vi "总氮通讯.vi"() -> ()   [LabVIEW 2016, in "斯坦道总氮.lvlib"]
uses:
  <vilib>/Plasmionique/MB Master/MB_Master_TCP/MB_Master_TCP.lvclass
  C:/Program Files (x86)/National Instruments/LabVIEW 2016/vi.lib/Plasmionique/MB Master/MB_Master/MB_Master.lvclass
  <vilib>/NI/Modbus Library/API/Wrapper/Create TCP Slave.vi
  <vilib>/Utility/config.llb/Write Key (Boolean).vi
  <vilib>/Utility/config.llb/Write Key (String).vi
  <vilib>/Plasmionique/MB Master/MB_Master/MB_Master.lvclass
  <vilib>/NI/Modbus Library/API/slave/Modbus Slave.lvclass
  <vilib>/Utility/config.llb/NI_LVConfig.lvlib
  <vilib>/Plasmionique/MB Master/MB Master.lvlib
  <vilib>/NI/Modbus Library/API/Wrapper/API Main.lvlib
panel:
  out "总氮测量数据区":u16[](array[numeric])
  out "总氮状态告警区":u16[](array[numeric])
  out "总磷状态告警区":u16[](array[numeric])
  out "总磷测量数据区":u16[](array[numeric])
  out "序列号":string
  out "状态告警区":T1
  out "测量数据区":T2 {"单位" items=["ug/L", "mg/L", "ppm", "mg/m3", "cm", "ppb", "ug/m3", "%", "nmol/mol", "umol/mol", "MPN/L", "MPN/100ml", "ng/m3", "NTU", "无量纲", "ms/cm", "us/cm", "℃", "mV", "万个/L"]}
  out "status":bool
  out "关键参数区":T3
  in  "读关键参数区":bool
  in  "读状态告警区":bool
  in  "读测量数据区":bool
  in  "站号":u16(ring) items=["总磷"=1, "氨氮"=3]
  in  "停止":bool
  in  "启动":bool
  in  "控制命令":u16(ring) items=["启动测量"=1, "标样核查"=2, "零点核查"=3, "跨度核查"=4, "空白测试"=5, "平行样测试"=6, "加标回收"=7, "空白校准"=8, "标样校准"=9, "初始化（清洗）"=10, "停止测试"=11, "仪器重启"=12, "校时"=13, "模式设置"=14, "测量间隔设置"=15]
  in  "控制命令参数":u16[](array[numeric]) format="%04xH"
  in  "VISA Resource":refnum<visa-resource-name>
  in  "启用模块":bool
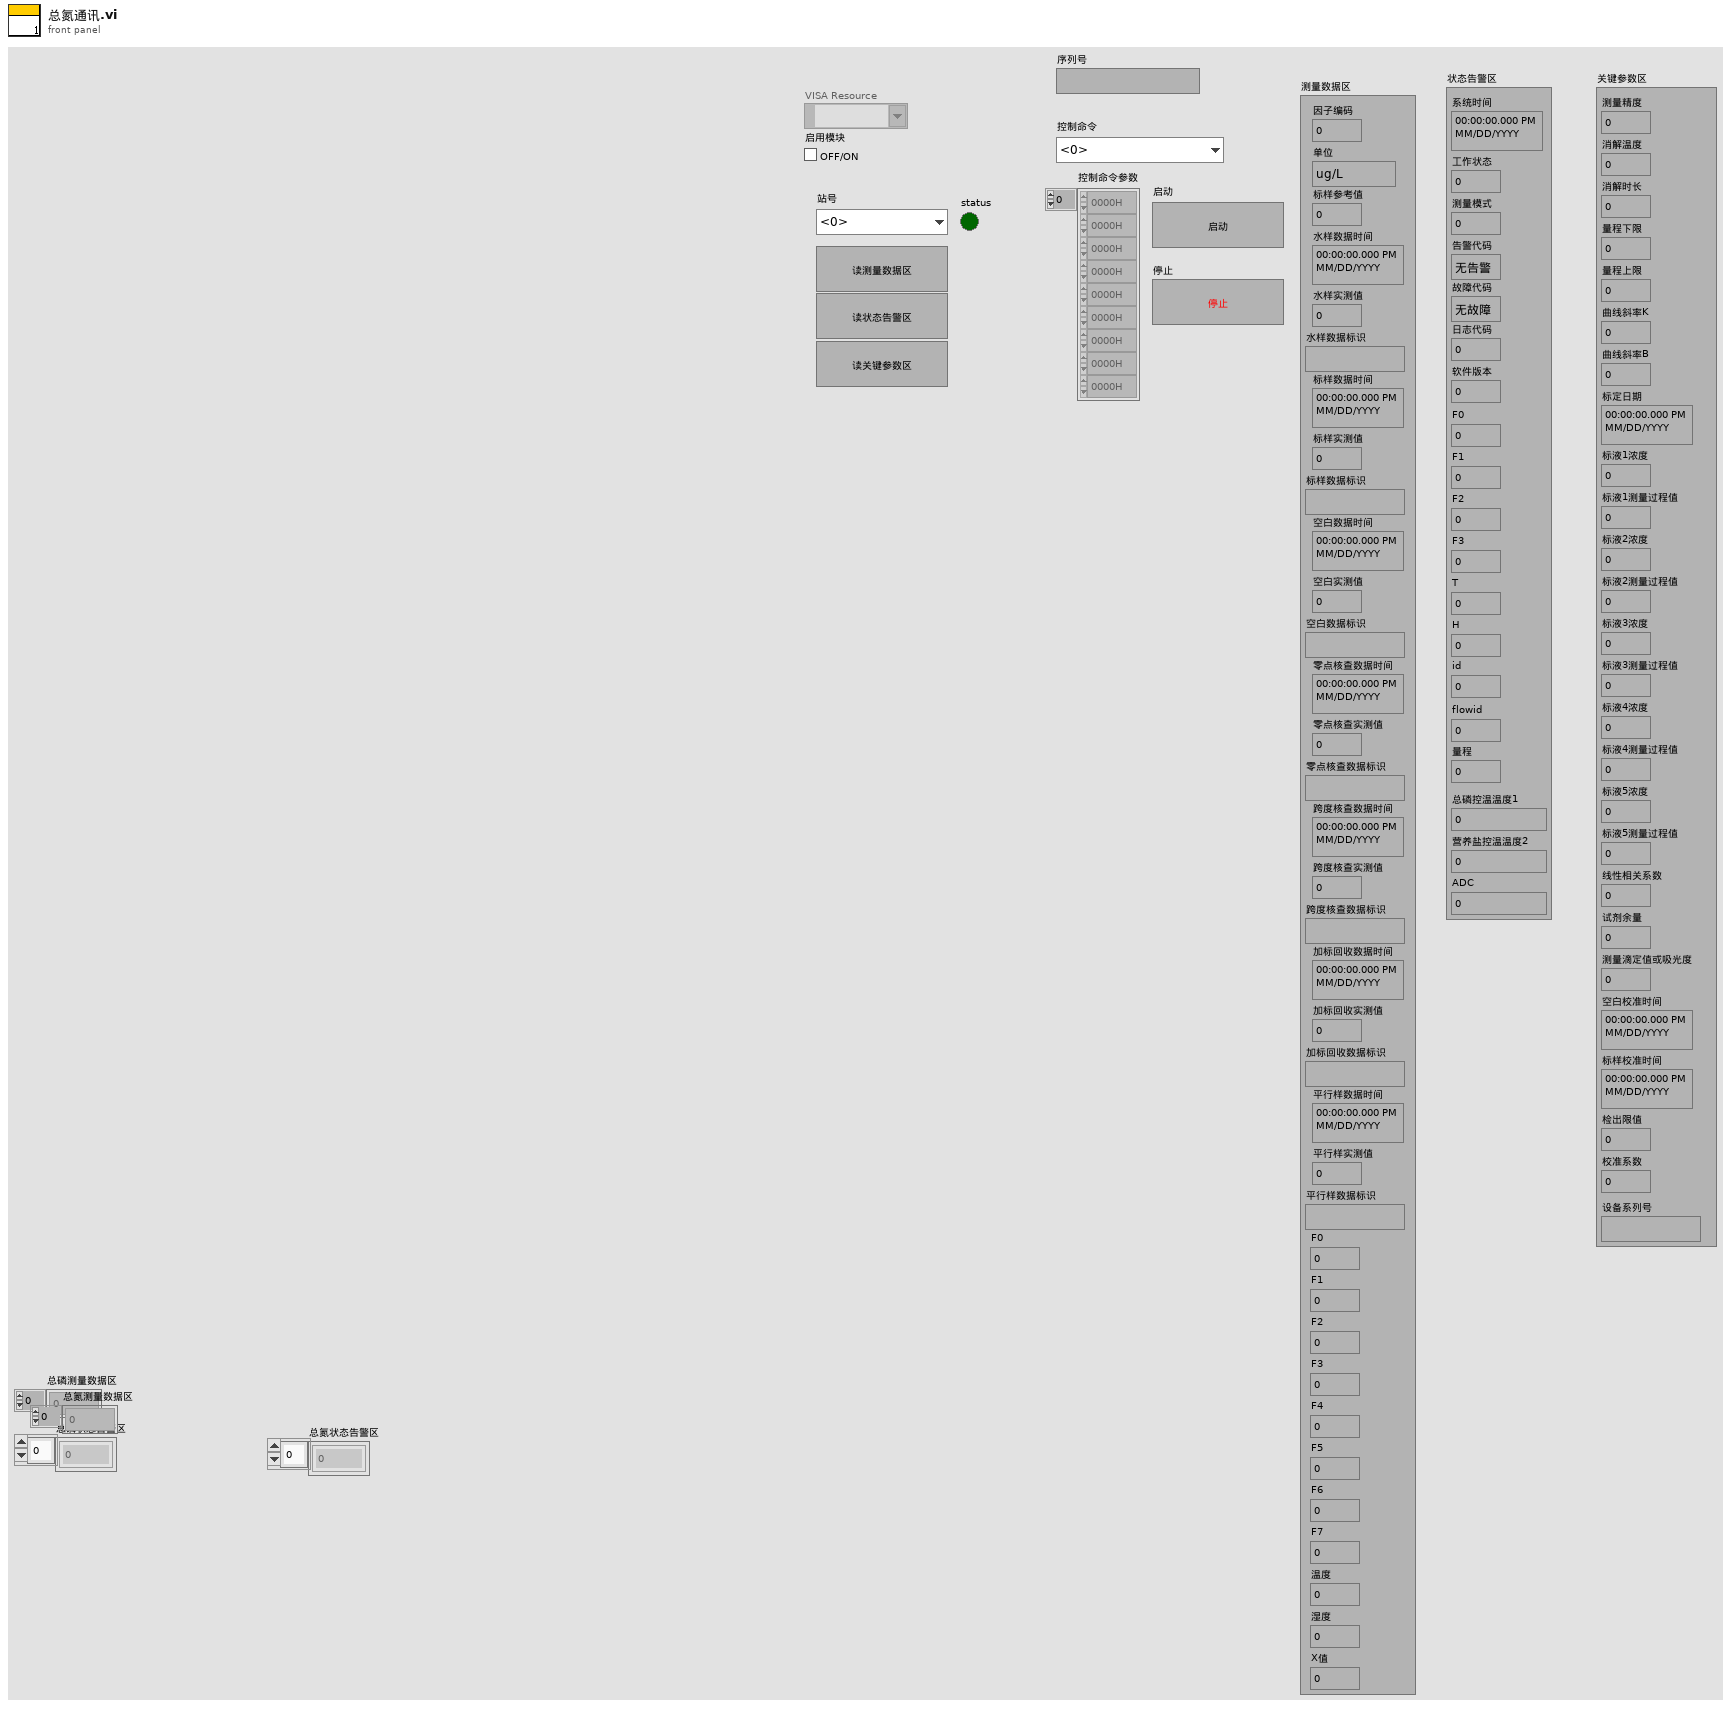
[diagram p1: front panel]
types:
  T1 = cluster{"系统时间":timestamp, "工作状态":u16, "测量模式":u16, "告警代码":enum16{"无告警", "缺试剂告警", "缺水样告警", "缺蒸馏水告警", "缺标液告警", "仪表漏液告警", "标定异常告警", "超量程告警", "加热异常", "低试剂预警", "超上限告警", "超下限告警", "仪表内部其他异常", "滴定异常告警", "电极异常告警", "量程切换告警", "参数设置告警", "PH电极电位异常", "电导率电极异常", "浊度光度异常", "溶解氧电极异常", "溶解氧光强异常", "温度异常告警", "PH异常告警", "溶解氧异常告警", "电导率异常告警", "浊度异常告警", "叶绿素异常告警", "藻密度异常告警", "蓝绿藻异常告警", "ORP异常告警", "氨氮异常告警", "清洁刷异常告警", "SD卡异常告警", "蓝牙异常告警", "Wifi异常告警", "流程异常告警"}, "故障代码":enum16{"无故障", "电机故障", "温度故障", "通讯故障", "滴定故障"}, "日志代码":u16, "软件版本":u16, "F0":sgl, "F1":sgl, "F2":sgl, "F3":sgl, "T":sgl, "H":sgl, "id":u16, "flowid":u16, "量程":u16, "总磷控温温度1":sgl, "营养盐控温温度2":sgl, "ADC":sgl}
  T2 = cluster{"因子编码":u32, "单位":u16, "标样参考值":sgl, "水样数据时间":timestamp, "水样实测值":sgl, "水样数据标识":string, "标样数据时间":timestamp, "标样实测值":sgl, "标样数据标识":string, "空白数据时间":timestamp, "空白实测值":sgl, "空白数据标识":string, "零点核查数据时间":timestamp, "零点核查实测值":sgl, "零点核查数据标识":string, "跨度核查数据时间":timestamp, "跨度核查实测值":sgl, "跨度核查数据标识":string, "加标回收数据时间":timestamp, "加标回收实测值":sgl, "加标回收数据标识":string, "平行样数据时间":timestamp, "平行样实测值":sgl, "平行样数据标识":string, "F0":sgl, "F1":sgl, "F2":sgl, "F3":sgl, "F4":sgl, "F5":sgl, "F6":sgl, "F7":sgl, "温度":sgl, "湿度":sgl, "X值":sgl}
  T3 = cluster{"测量精度":u16, "消解温度":u16, "消解时长":u16, "量程下限":sgl, "量程上限":sgl, "曲线斜率K":sgl, "曲线斜率B":sgl, "标定日期":timestamp, "标液1浓度":sgl, "标液1测量过程值":sgl, "标液2浓度":sgl, "标液2测量过程值":sgl, "标液3浓度":sgl, "标液3测量过程值":sgl, "标液4浓度":sgl, "标液4测量过程值":sgl, "标液5浓度":sgl, "标液5测量过程值":sgl, "线性相关系数":sgl, "试剂余量":u32, "测量滴定值或吸光度":sgl, "空白校准时间":timestamp, "标样校准时间":timestamp, "检出限值":sgl, "校准系数":sgl, "设备系列号":string}
  T4 = typedef "NI_LVConfig.lvlib/Config Data RefNum.ctl" = refnum<k1>
  T5 = enum8{"Enabled", "Disabled", "Disabled and Grayed Out"}
  T6 = cluster{"系统时间":timestamp, "工作状态":enum16{"空闲", "水样测试", "标样核查", "零点核查", "跨度核查", "空白测试", "平行样测试", "加标回收", "空白校准", "标样校准", "初始化（清洗）"}, "测量模式":enum16{"待机", "连续模式", "周期模式", "定点模式", "受控模式", "手动模式"}, "告警代码":enum16{"无告警", "缺试剂告警", "缺水样告警", "缺蒸馏水告警", "缺标液告警", "仪表漏液告警", "标定异常告警", "超量程告警", "加热异常", "低试剂预警", "超上限告警", "超下限告警", "仪表内部其他异常", "滴定异常告警", "电极异常告警", "量程切换告警", "参数设置告警", "PH电极电位异常", "电导率电极异常", "浊度光度异常", "溶解氧电极异常", "溶解氧光强异常", "温度异常告警", "PH异常告警", "溶解氧异常告警", "电导率异常告警", "浊度异常告警", "叶绿素异常告警", "藻密度异常告警", "蓝绿藻异常告警", "ORP异常告警", "氨氮异常告警", "清洁刷异常告警", "SD卡异常告警", "蓝牙异常告警", "Wifi异常告警", "流程异常告警"}, "故障代码":enum16{"无故障", "电机故障", "温度故障", "通讯故障", "滴定故障"}, "日志代码":u16, "软件版本":u16, "F0":sgl, "F1":sgl, "F2":sgl, "F3":sgl, "T":sgl, "H":sgl, "id":u16, "flowid":u16, "量程":u16, "总磷控温温度1":sgl, "营养盐控温温度2":sgl, "ADC":sgl}
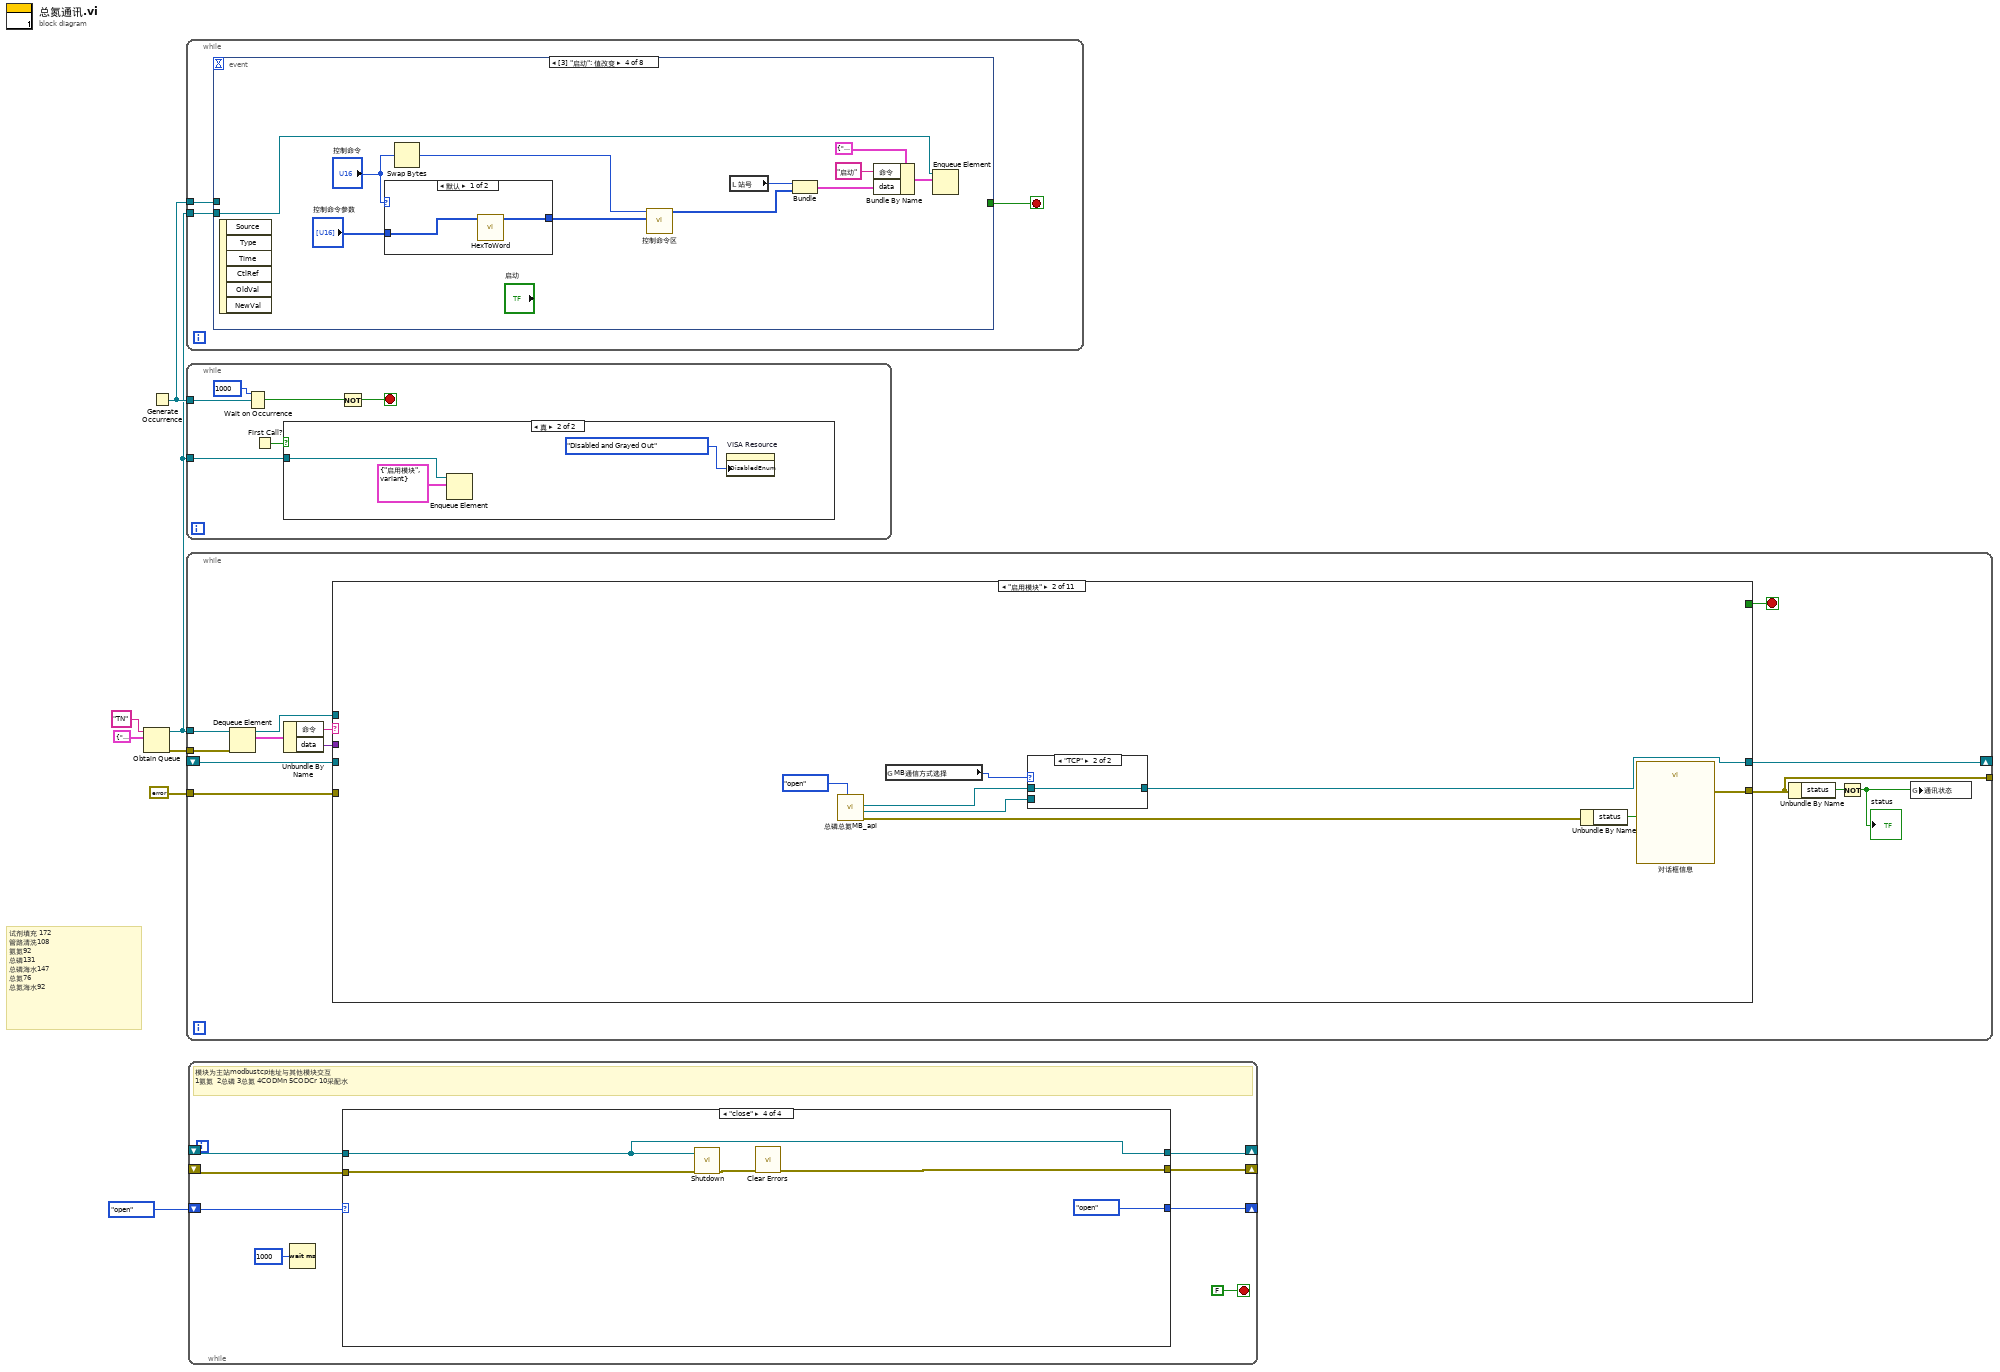
[diagram p0: block diagram]
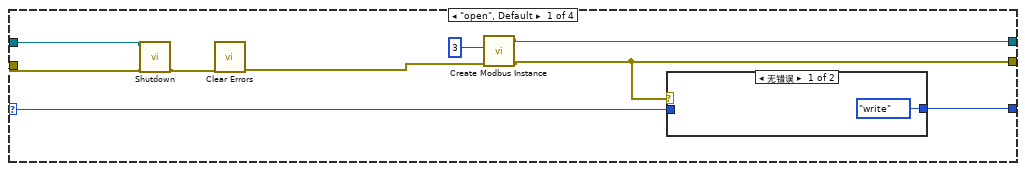
[diagram p2: hidden frame]
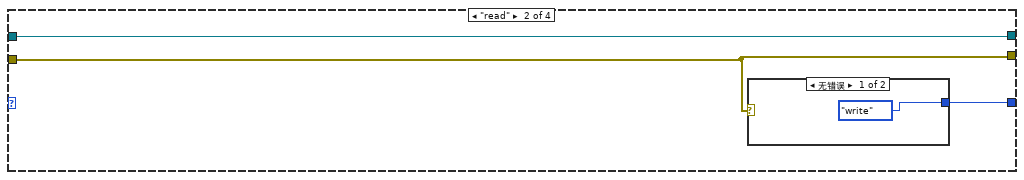
[diagram p4: hidden frame]
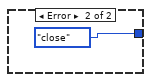
[diagram p5: hidden frame]
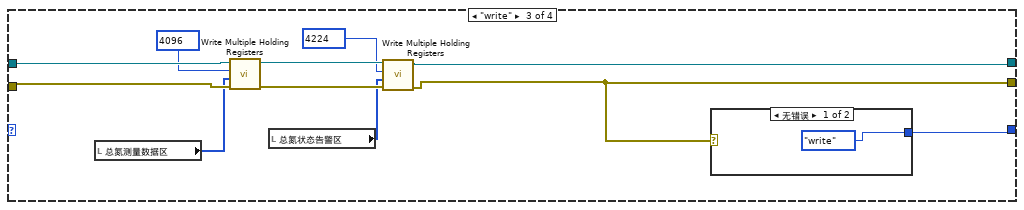
[diagram p6: hidden frame]
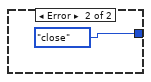
[diagram p7: hidden frame]
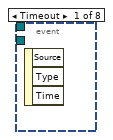
[diagram p9: hidden frame]
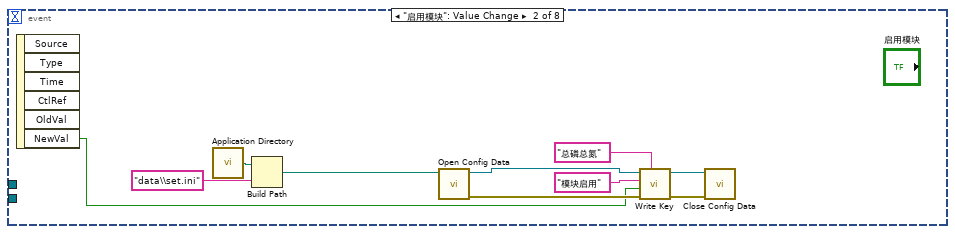
[diagram p10: hidden frame]
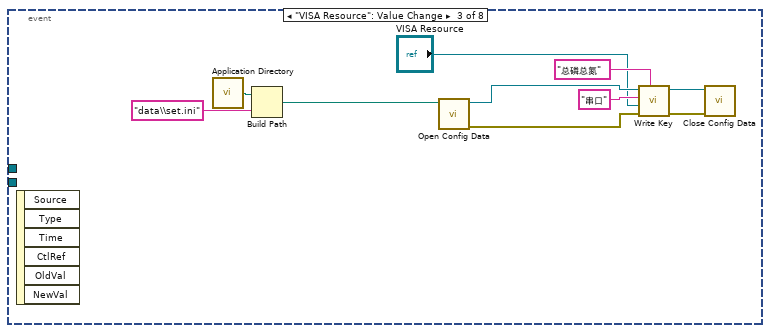
[diagram p11: hidden frame]
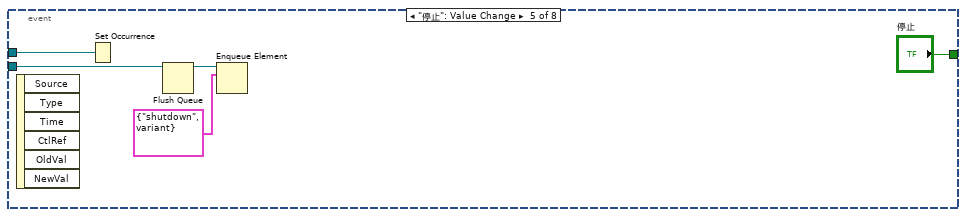
[diagram p13: hidden frame]
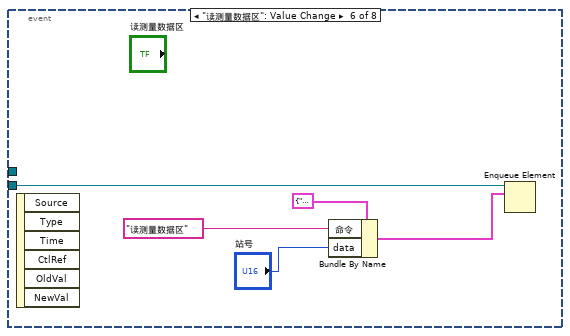
[diagram p14: hidden frame]
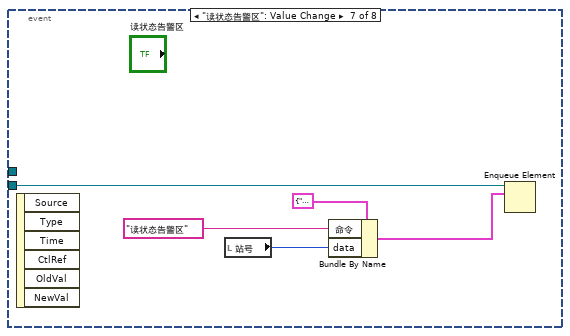
[diagram p15: hidden frame]
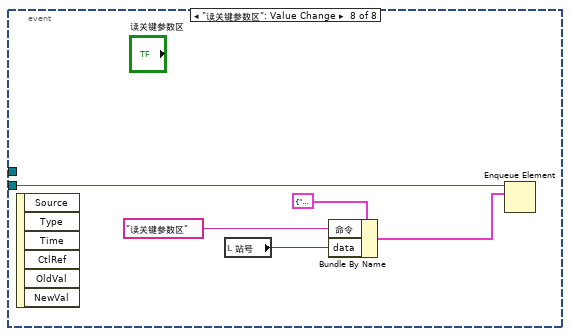
[diagram p16: hidden frame]
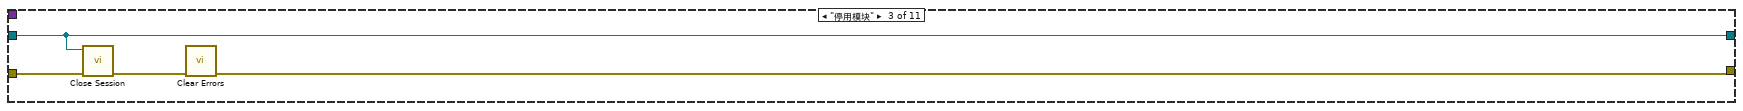
[diagram p19: hidden frame]
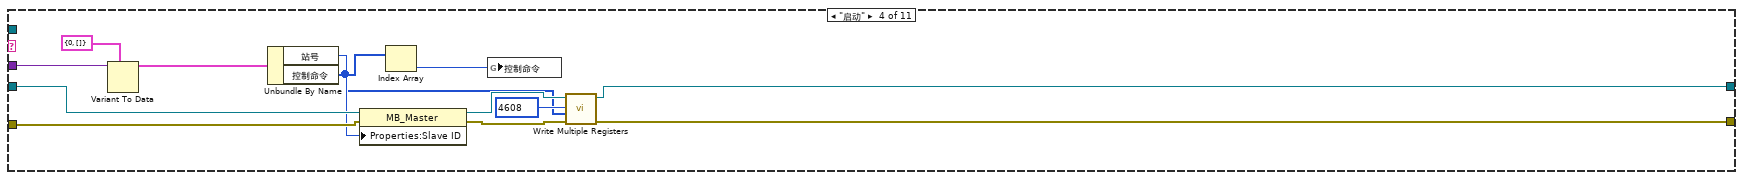
[diagram p20: hidden frame]
diagram:
  # "试剂填充 172 \n管路清洗108\n氨氮92\n总磷131\n总磷海水147\n总氮76\n总氮海水92"
  n1 = Obtain Queue(name (unnamed)="TN" ("名称（未命名）"), element data type=cluster{"命令":string, "data":variant} {"命令"="", "data"=variant}) -> (queue out=w2:refnum<queue>, error out=w5:errorcluster)  [unwired: 3 in, 1 out]
  n2 = Generate Occurrence() -> (w3:refnum<k4>)
  n3 = while {
    tunnel: w2 -> [w10]
    tunnel: w3 -> [w8]
    stop <- w9 stop-if-true
    n4 = event shown="[3] \"启动\": 值改变" {
      selector: _ -> [_ _ _ _ _ _ _ _]
      dyn-events: _ -> [_ _ _ _ _ _ _ _]
      timeout: _ -> [_ _ _ _ _ _ _ _]
      tunnel: w10 -> [_ _ _ w41 w48 w54 w59 w64]
      tunnel: [_ _ _ _ "停止" _ _ _] -> w9
      tunnel: w8 -> [_ _ _ _ w45 _ _ _]
      event Timeout {
        n5 = event-data() -> ()  [unwired: 1 in, 3 out]
      }
      event "启用模块": Value Change {
        n6 = event-data() -> ("NewVal"=w11:bool)  [unwired: 1 in, 5 out]
        n7 = call <vilib>:"Application Directory.vi"() -> ("Application Directory"=w13:path)
        n8 = Build Path(base path=w13, name or relative path="data\\set.ini" ("名称或相对路径")) -> (appended path=w14:path)
        n9 = call <vilib>:"Open Config Data.vi"("configuration file path"=w14) -> ("error out"=w20:errorcluster, "refnum"=w19:T4)  [unwired: 8 in, 1 out]
        n10 = call-poly <vilib>:"Write Key.vi"("section"="总磷总氮", "error in (no error)"=w20, "value"=w11, "key"="模块启用", "refnum"=w19) -> ("error out"=w16:errorcluster, "refnum out"=w12:T4)  [unwired: 4 in, 1 out]
        n11 = call <vilib>:"Close Config Data.vi"("error in (no error)"=w16, "refnum"=w12) -> ()  [unwired: 8 in, 2 out]
      }
      event "VISA Resource": Value Change {
        n12 = event-data() -> ()  [unwired: 1 in, 6 out]
        n13 = call <vilib>:"Application Directory.vi"() -> ("Application Directory"=w23:path)
        n14 = Build Path(base path=w23, name or relative path="data\\set.ini" ("名称或相对路径")) -> (appended path=w24:path)
        n15 = call <vilib>:"Open Config Data.vi"("configuration file path"=w24) -> ("error out"=w30:errorcluster, "refnum"=w29:T4)  [unwired: 8 in, 1 out]
        n16 = call-poly <vilib>:"Write Key.vi"("section"="总磷总氮", "error in (no error)"=w30, "value"="VISA Resource", "key"="串口", "refnum"=w29) -> ("error out"=w26:errorcluster, "refnum out"=w22:T4)  [unwired: 4 in, 1 out]
        n17 = call <vilib>:"Close Config Data.vi"("error in (no error)"=w26, "refnum"=w22) -> ()  [unwired: 8 in, 2 out]
      }
      event "启动": Value Change {
        n18 = event-data() -> ()  [unwired: 1 in, 6 out]
        n19 = case shown="默认" "控制命令" {
          tunnel: "控制命令参数" -> [w43 w44]
          tunnel: [w42 w44] -> w31
          frame Default {
            n20 = call "HexToWord.vi"("数组"=w43) -> ("WORD"=w42:u16[])  [unwired: 10 in]
          }
          frame 13 {
          }
        }
        n21 = Swap Bytes(anything="控制命令") -> (byte swapped=w34:u16)
        n22 = call "控制命令区.vi"("控制命令参数"=w31, "控制命令"=w34) -> ("控制命令"=w37:u16[])  [unwired: 9 in]
        n23 = local read "站号"() -> (w36:u16)
        n24 = Bundle("站号"=w36, "控制命令"=w37) -> (w35:cluster{"站号":u16, "控制命令":u16[]})  [unwired: 1 in]
        n25 = Bundle By Name(cluster=cluster{"命令":string, "data":variant} {"命令"="", "data"=variant} ("元素"), "命令"="启动", "data"=w35) -> (w39:cluster{"命令":string, "data":variant})
        n26 = Enqueue Element(queue=w41, element=w39) -> ()  [unwired: 2 in, 3 out]
      }
      event "停止": Value Change {
        n27 = event-data() -> ()  [unwired: 1 in, 6 out]
        n28 = Set Occurrence(w45) -> ()
        n29 = Flush Queue(queue=w48) -> (queue out=w47:refnum<queue>)  [unwired: 1 in, 2 out]
        n30 = Enqueue Element(queue=w47, element=cluster{"命令":string, "data":variant} {"命令"="shutdown", "data"=variant} ("元素")) -> ()  [unwired: 2 in, 3 out]
      }
      event "读测量数据区": Value Change {
        n31 = event-data() -> ()  [unwired: 1 in, 6 out]
        n32 = Bundle By Name(cluster=cluster{"命令":string, "data":variant} {"命令"="", "data"=variant} ("元素"), "命令"="读测量数据区", "data"="站号") -> (w52:cluster{"命令":string, "data":variant})
        n33 = Enqueue Element(queue=w54, element=w52) -> ()  [unwired: 2 in, 3 out]
      }
      event "读状态告警区": Value Change {
        n34 = event-data() -> ()  [unwired: 1 in, 6 out]
        n35 = local read "站号"() -> (w55:u16)
        n36 = Bundle By Name(cluster=cluster{"命令":string, "data":variant} {"命令"="", "data"=variant} ("元素"), "命令"="读状态告警区", "data"=w55) -> (w57:cluster{"命令":string, "data":variant})
        n37 = Enqueue Element(queue=w59, element=w57) -> ()  [unwired: 2 in, 3 out]
      }
      event "读关键参数区": Value Change {
        n38 = event-data() -> ()  [unwired: 1 in, 6 out]
        n39 = local read "站号"() -> (w60:u16)
        n40 = Bundle By Name(cluster=cluster{"命令":string, "data":variant} {"命令"="", "data"=variant} ("元素"), "命令"="读关键参数区", "data"=w60) -> (w62:cluster{"命令":string, "data":variant})
        n41 = Enqueue Element(queue=w64, element=w62) -> ()  [unwired: 2 in, 3 out]
      }
    }
  }
  n42 = while {
    tunnel: w3 -> [w70]
    tunnel: w2 -> [w66]
    stop <- w67 stop-if-true
    n43 = Wait on Occurrence(2:w70, 3:1000 ("毫秒超时(-1)")) -> (0:w68:bool)  [unwired: 1 in]
    n44 = First Call?() -> (First Call?: T/F=w65:bool)
    n45 = case shown="真" w65 {
      tunnel: w66 -> [_ w72]
      frame False {
      }
      frame True {
        n46 = Enqueue Element(queue=w72, element=cluster{"命令":string, "data":variant} {"命令"="启用模块", "data"=variant} ("元素")) -> ()  [unwired: 2 in, 3 out]
        n47 = property on="VISA Resource" class="VISAName"("DisabledEnum"=T5."Disabled and Grayed Out" ("禁用")) -> ()  [unwired: 2 in, 2 out]
      }
    }
    n48 = Not(x=w68) -> (.not. x?=w67:bool)
  }
  n49 = while {
    tunnel: w2 -> [w86]
    tunnel: w5 -> [w85]
    shift-right: [w83] -> _
    shift-left: _ -> [w82]
    tunnel: errorcluster {"status"=FALSE, "code"=0, "source"=""} ("error out") -> [w81]
    tunnel: [w76] -> _
    stop <- w84 stop-if-true
    n50 = Dequeue Element(queue=w86, error in (no error)=w85) -> (queue out=w77:refnum<queue>, element=w79:cluster{"命令":string, "data":variant})  [unwired: 1 in, 2 out]
    n51 = Unbundle By Name(w79) -> ("命令"=w80:string, "data"=w78:variant)
    n52 = case shown="\"启用模块\"" w80 {
      tunnel: w78 -> [_ _ _ w112 w123 w140 w150 w164 w182 w196 _]
      tunnel: w77 -> [_ _ _ _ _ _ _ _ _ _ w209]
      tunnel: [_ _ _ _ _ _ _ _ _ _ TRUE] -> w84
      tunnel: [w87 w89 w99 w115 w126 w142 w154 w173 w189 w203 w205] -> w83
      tunnel: [w88 w95 w100 w114 w125 w141 w155 w163 w190 w204 w206] -> w76
      tunnel: w82 -> [w87 _ w99 w111 w122 w139 w149 w167 w185 w199 w205]
      tunnel: w81 -> [w88 _ w102 w108 w119 w136 w147 w168 w186 w200 w207]
      frame Default {
      }
      frame "启用模块" {
        n53 = call "总磷总氮MB_api.vi"("STEP"=enum16{"open", "read", "write", "close"}."open") -> ("error out"=w93:errorcluster, "MB session out"=w90:refnum<class "MB_Master.lvclass">, "MB_TCP session"=w91:refnum<class "MB_Master_TCP.lvclass">)  [unwired: 7 in, 1 out]
        n54 = global read "总氮断电保存全局变量.vi" "MB通信方式选择"() -> (w92:enum16{"串口", "TCP"})
        n55 = case shown="\"TCP\"" w92 {
          tunnel: w91 -> [_ w98]
          tunnel: w90 -> [w97 _]
          tunnel: [w97 w98] -> w89
          frame "串口", Default {
          }
          frame "TCP" {
          }
        }
        n56 = Unbundle By Name(w93) -> ("status"=w96:bool)
        n57 = call "对话框信息"("Enable"=w96) -> ("error out"=w95:errorcluster)  [unwired: 9 in, 1 out]
      }
      frame "停用模块" {
        n58 = call-dynamic "Close Session.vi"("error in (no error)"=w102, "MB session in"=w99) -> ("error out"=w101:errorcluster)  [unwired: 9 in]
        n59 = call <vilib>:"Clear Errors.vi"("error in (no error)"=w101) -> ("error out"=w100:errorcluster)  [unwired: 5 in, 1 out]
      }
      frame "启动" {
        n60 = Variant To Data(type=cluster{"站号":u16, "控制命令":u16[]} {"站号"=0, "控制命令"=[]} ("输出簇"), Variant=w112) -> (data=w106:cluster{"站号":u16, "控制命令":u16[]})  [unwired: 1 in, 1 out]
        n61 = Unbundle By Name(w106) -> ("站号"=w105:u16, "控制命令"=w103:u16[])
        n62 = property class="MB_Master"(reference=w111, error in=w108, "Properties:Slave ID"=w105) -> (reference out=w110:refnum<class "MB_Master.lvclass">, error out=w109:errorcluster)
        n63 = Index Array(array=w103) -> (element=w104:u16)  [unwired: 1 in]
        n64 = global write "VAR总氮全局变量.vi" "控制命令"(w104) -> ()
        n65 = call <vilib>:"Write Multiple Registers.vi"("error in (no error)"=w109, "values"=w103, "starting address"=u16 4608, "MB session in"=w110) -> ("error out"=w114:errorcluster, "MB session out"=w115:refnum<class "MB_Master.lvclass">)  [unwired: 6 in]
      }
      frame "盲样测试" {
        n66 = Variant To Data(type=0, Variant=w123) -> (data=w116:i32)  [unwired: 1 in, 1 out]
        n67 = case shown="默认" w116 {
          tunnel: [u16[] [] ("values") u16[] [33539, 0] ("values") u16[] [23555, 0] ("values")] -> w118
          frame Default {
          }
          frame 1 {
            # "总磷盲样测试命令"
          }
          frame 3 {
            # "氨氮盲样测试"
          }
        }
        n68 = property class="MB_Master"(reference=w122, error in=w119, "Properties:Slave ID"=w116) -> (reference out=w121:refnum<class "MB_Master.lvclass">, error out=w120:errorcluster)
        n69 = call <vilib>:"Write Multiple Registers.vi"("error in (no error)"=w120, "values"=w118, "starting address"=u16 24592, "MB session in"=w121) -> ("error out"=w125:errorcluster, "MB session out"=w126:refnum<class "MB_Master.lvclass">)  [unwired: 6 in]
      }
      frame "debug" {
        n70 = Variant To Data(type=cluster{"站号":u16, "控制命令":u16[]} {"站号"=0, "控制命令"=[]} ("输出簇"), Variant=w140) -> (data=w134:cluster{"站号":u16, "控制命令":u16[]})  [unwired: 1 in, 1 out]
        n71 = Unbundle By Name(w134) -> ("站号"=w133:u16, "控制命令"=w131:u16[])
        n72 = property class="MB_Master"(reference=w139, error in=w136, "Properties:Slave ID"=w133) -> (reference out=w138:refnum<class "MB_Master.lvclass">, error out=w137:errorcluster)
        n73 = Index Array(array=w131) -> (element=w132:u16)  [unwired: 1 in]
        n74 = global write "VAR总氮全局变量.vi" "控制命令"(w132) -> ()
        n75 = call <vilib>:"Write Multiple Registers.vi"("error in (no error)"=w137, "values"=w131, "starting address"=u16 24594, "MB session in"=w138) -> ("error out"=w141:errorcluster, "MB session out"=w142:refnum<class "MB_Master.lvclass">)  [unwired: 6 in]
      }
      frame "读测量数据区" {
        n76 = Variant To Data(type=u8 1 ("Slave ID"), Variant=w150) -> (data=w145:u8)  [unwired: 1 in, 1 out]
        n77 = property class="MB_Master"(reference=w149, error in=w147, "Properties:Slave ID"=w145) -> (reference out=w148:refnum<class "MB_Master.lvclass">, error out=w146:errorcluster)
        n78 = call <vilib>:"Read Holding Registers.vi"("error in (no error)"=w146, "quantity"=u16 104, "starting address"=u16 4096, "MB session in"=w148) -> ("error out"=w155:errorcluster, "Registers"=w144:u16[], "MB session out"=w154:refnum<class "MB_Master.lvclass">)  [unwired: 5 in]
        n79 = call "测量数据区.vi"("数组"=w144) -> ("测量数据区"=w143:T2)  [unwired: 10 in]
        "测量数据区" <- w143
        n80 = case shown="2" w145 {
          tunnel: w143 -> [_ w156 w158]
          tunnel: w144 -> [_ w157 w159]
          frame 0, Default {
          }
          frame 1 {
            n81 = global write "VAR总氮全局变量.vi" "总磷测量数据区"(w156) -> ()
            "总磷测量数据区" <- w157
          }
          frame 2 {
            n82 = global write "VAR总氮全局变量.vi" "总氮测量数据区"(w158) -> ()
            "总氮测量数据区" <- w159
          }
        }
        n83 = global write "VAR总氮全局变量.vi" "测量数据区"(w143) -> ()
      }
      frame "读状态告警区" {
        n84 = Variant To Data(type=u8 1 ("Slave ID"), Variant=w164) -> (data=w169:u8)  [unwired: 1 in, 1 out]
        n85 = property class="MB_Master"(reference=w167, error in=w168, "Properties:Slave ID"=w169) -> (reference out=w166:refnum<class "MB_Master.lvclass">, error out=w165:errorcluster)
        n86 = call <vilib>:"Read Holding Registers.vi"("error in (no error)"=w165, "quantity"=u16 29, "starting address"=u16 4224, "MB session in"=w166) -> ("error out"=w163:errorcluster, "Registers"=w160:u16[], "MB session out"=w173:refnum<class "MB_Master.lvclass">)  [unwired: 5 in]
        n87 = call "状态告警区.vi"("数组"=w160) -> ("状态告警区"=w161:T6)  [unwired: 10 in]
        "状态告警区" <- w161
        n88 = global write "VAR总氮全局变量.vi" "状态告警区"(w161) -> ()
        n89 = Unbundle By Name(w161) -> ("id"=w162:u16)
        n90 = case shown="2, 76" w162 {
          tunnel: w161 -> [_ w174 w176]
          tunnel: w160 -> [_ w175 w177]
          frame 0, Default {
          }
          frame 1, 131 {
            n91 = global write "VAR总氮全局变量.vi" "总磷状态告警区"(w174) -> ()
            "总磷状态告警区" <- w175
          }
          frame 2, 76 {
            n92 = global write "VAR总氮全局变量.vi" "总氮状态告警区"(w176) -> ()
            "总氮状态告警区" <- w177
          }
        }
      }
      frame "读关键参数区" {
        n93 = Variant To Data(type=u8 1 ("Slave ID"), Variant=w182) -> (data=w180:u8)  [unwired: 1 in, 1 out]
        n94 = property class="MB_Master"(reference=w185, error in=w186, "Properties:Slave ID"=w180) -> (reference out=w184:refnum<class "MB_Master.lvclass">, error out=w183:errorcluster)
        n95 = call <vilib>:"Read Holding Registers.vi"("error in (no error)"=w183, "quantity"=u16 19, "starting address"=u16 4256, "MB session in"=w184) -> ("error out"=w190:errorcluster, "Registers"=w179:u16[], "MB session out"=w189:refnum<class "MB_Master.lvclass">)  [unwired: 5 in]
        n96 = call "关键参数区.vi"("数组"=w179) -> ("关键参数区"=w178:T3)  [unwired: 10 in]
        "关键参数区" <- w178
        n97 = global write "VAR总氮全局变量.vi" "关键参数区"(w178) -> ()
      }
      frame "读序列号" {
        n98 = Variant To Data(type=u8 1 ("Slave ID"), Variant=w196) -> (data=w194:u8)  [unwired: 1 in, 1 out]
        n99 = property class="MB_Master"(reference=w199, error in=w200, "Properties:Slave ID"=w194) -> (reference out=w198:refnum<class "MB_Master.lvclass">, error out=w197:errorcluster)
        n100 = call <vilib>:"Read Holding Registers.vi"("error in (no error)"=w197, "quantity"=u16 6, "starting address"=u16 3, "MB session in"=w198) -> ("error out"=w204:errorcluster, "Registers"=w193:u16[], "MB session out"=w203:refnum<class "MB_Master.lvclass">)  [unwired: 5 in]
        n101 = call "HexToString.vi"("数组"=w193) -> ("STRING"=w192:string[])  [unwired: 10 in]
        n102 = Index Array(array=w192) -> (element=w191:string)  [unwired: 1 in]
        "序列号" <- w191
        n103 = global write "VAR总氮全局变量.vi" "序列号"(w191) -> ()
      }
      frame "shutdown" {
        n104 = call-dynamic "Close Session.vi"("error in (no error)"=w207, "MB session in"=w205) -> ("error out"=w206:errorcluster)  [unwired: 9 in]
        n105 = Flush Queue(queue=w209) -> (queue out=w208:refnum<queue>)  [unwired: 1 in, 2 out]
        n106 = Release Queue(queue=w208) -> ()  [unwired: 2 in, 3 out]
      }
    }
    n107 = Unbundle By Name(w76) -> ("status"=w75:bool)
    n108 = Not(x=w75) -> (.not. x?=w74:bool)
    "status" <- w74
    n109 = global write "VAR总氮全局变量.vi" "通讯状态"(w74) -> ()
  }
  n110 = while {
    shift-right: [w216] -> _
    shift-left: _ -> [w218]
    shift-right: [w215] -> _
    shift-left: _ -> [w217]
    shift-right: [w212] -> _
    shift-left: enum16{"open", "read", "write", "close"}."open" -> [w213]
    stop <- FALSE stop-if-true
    # "模块为主站modbustcp地址与其他模块交互\n1氨氮  2总磷 3总氮 4CODMn 5CODCr 10采配水"
    n111 = Wait (ms)(milliseconds to wait=u32 1000 ("等待时间（毫秒）")) -> ()  [unwired: 1 out]
    n112 = case shown="\"close\"" w213 {
      selector: w213 -> [w227 _ _ _]
      tunnel: w218 -> [w221 w230 w244 w250]
      tunnel: w217 -> [w220 w231 w243 w249]
      tunnel: [w224 w230 w239 w250] -> w216
      tunnel: [w223 w231 w238 w252] -> w215
      tunnel: [w226 w232 w245 enum16{"open", "read", "write", "close"}."open"] -> w212
      frame "open", Default {
        n113 = call-dynamic "Shutdown.vi"("error in"=w220, "Modbus slave in"=w221) -> ("error out"=w219:errorcluster)  [unwired: 9 in]
        n114 = call <vilib>:"Clear Errors.vi"("error in (no error)"=w219) -> ("error out"=w222:errorcluster)  [unwired: 5 in, 1 out]
        n115 = call-poly <vilib>:"Create Modbus Instance.vi"("error in"=w222, "port (502)"=u16 3) -> ("error out"=w223:errorcluster, "TCP slave instance"=w224:refnum<class "Modbus Slave.lvclass">)  [unwired: 8 in]
        n116 = case shown="无错误" w223 {
          tunnel: w227 -> [_ w229]
          tunnel: [enum16{"open", "read", "write", "close"}."write" w229] -> w226
          frame No Error {
          }
          frame Error {
          }
        }
      }
      frame "read" {
        n117 = case shown="无错误" w231 {
          tunnel: [enum16{"open", "read", "write", "close"}."write" enum16{"open", "read", "write", "close"}."close"] -> w232
          frame No Error {
          }
          frame Error {
          }
        }
      }
      frame "write" {
        n118 = local read "总氮测量数据区"() -> (w237:u16[])
        n119 = call-dynamic "Write Multiple Holding Registers.vi"("error in"=w243, "registers to write"=w237, "starting address"=u16 4096, "Modbus slave in"=w244) -> ("error out"=w240:errorcluster, "Modbus slave out"=w241:refnum<class "Modbus Slave.lvclass">)  [unwired: 6 in]
        n120 = local read "总氮状态告警区"() -> (w235:u16[])
        n121 = call-dynamic "Write Multiple Holding Registers.vi"("error in"=w240, "registers to write"=w235, "starting address"=u16 4224, "Modbus slave in"=w241) -> ("error out"=w238:errorcluster, "Modbus slave out"=w239:refnum<class "Modbus Slave.lvclass">)  [unwired: 6 in]
        n122 = case shown="无错误" w238 {
          tunnel: [enum16{"open", "read", "write", "close"}."write" enum16{"open", "read", "write", "close"}."close"] -> w245
          frame No Error {
          }
          frame Error {
          }
        }
      }
      frame "close" {
        n123 = call-dynamic "Shutdown.vi"("error in"=w249, "Modbus slave in"=w250) -> ("error out"=w248:errorcluster)  [unwired: 9 in]
        n124 = call <vilib>:"Clear Errors.vi"("error in (no error)"=w248) -> ("error out"=w252:errorcluster)  [unwired: 5 in, 1 out]
      }
    }
  }
